vi "MapAction.vi"(2 "error in (no error)":errorcluster, 3 "Action":enum16{"Remove", "Mark", "Clear All"}(ring), 4 "Id":string, 5 "EpiWrapper in":refnum<class "EpiWrapper.lvclass">) -> (0 "error out":errorcluster, 1 "EpiWrapper out":refnum<class "EpiWrapper.lvclass">)   [LabVIEW 2012, in "EpiWrapper.lvclass"]
uses:
  EpiWrapper.lvclass
  EpiWrapper.lvclass/EpiWrapper.ctl
  Controls/CurrentPad.ctl
  Controls/PadArea.ctl
  Controls/Pad.ctl
  Controls/SelectedPads.ctl
  PadLookupVar.vi
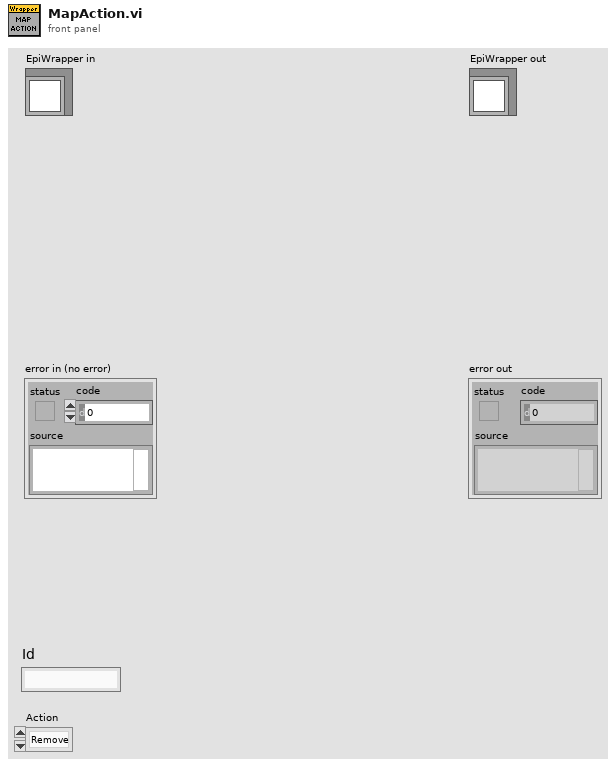
[diagram p1: front panel]
types:
  T1 = typedef "Pad.ctl" = cluster{"Coords":cluster{"Horizontal":sgl, "Vertical":sgl}, "radius":i32, "Tested":bool, "Selected":bool, "Id":string}
  T2 = typedef "MeasureControl.ctl" = cluster{"Graph":cluster{"Y":dbl[], "Y":dbl[]}[], "Pass":bool, "Fail":bool, "Measure":bool, "Wafer Area":T3, "TestData":T4, "Pad":string}
  T3 = typedef "PadArea.ctl" = enum16{"CenterA", "CenterB", "CenterC", "CenterD", "L", "R", "T", "G"}
  T4 = typedef "TestData.ctl" = cluster{"20mA Data":T5, "50mA Data ":T5}
  T5 = typedef "Measurement.ctl" = cluster{"Area":string, "Pad":string, "Current,mA":dbl, "Power":dbl, "WL":dbl, "Voltage":dbl, "Knee Current":dbl, "Reverse":dbl}
  T6 = typedef "SelectedPads.ctl" = T1[]
  T7 = typedef "CurrentPad.ctl" = cluster{"Coords":cluster{"Horizontal":sgl, "Vertical":sgl}, "radius":i32, "Tested":bool, "Selected":bool, "Pad":string, "PadArea":T8}
  T8 = typedef "PadArea.ctl" = enum16{"A", "B", "C", "D", "L", "R", "T", "G"}
  T9 = typedef "MapPOS.ctl" = cluster{"Coords":cluster{"Horizontal":sgl, "Vertical":sgl}, "radius":i32, "state":bool, "Id":string}[]
  T10 = typedef "PadLookup.ctl" = cluster{"A":T11, "B":T11, "C":T11, "D":T11, "L":T11, "R":T11, "T":T11, "G":T11}
  T11 = typedef "PadLookupItem.ctl" = cluster{"PadArea":T8, string[]}
  T12 = typedef "MeasureControl.ctl" = cluster{"Graph":cluster{"Y":dbl[], "Y":dbl[]}[], "Pass":bool, "Fail":bool, "Measure":bool, "Wafer Area":T8, "TestData":T4, "Pad":string}
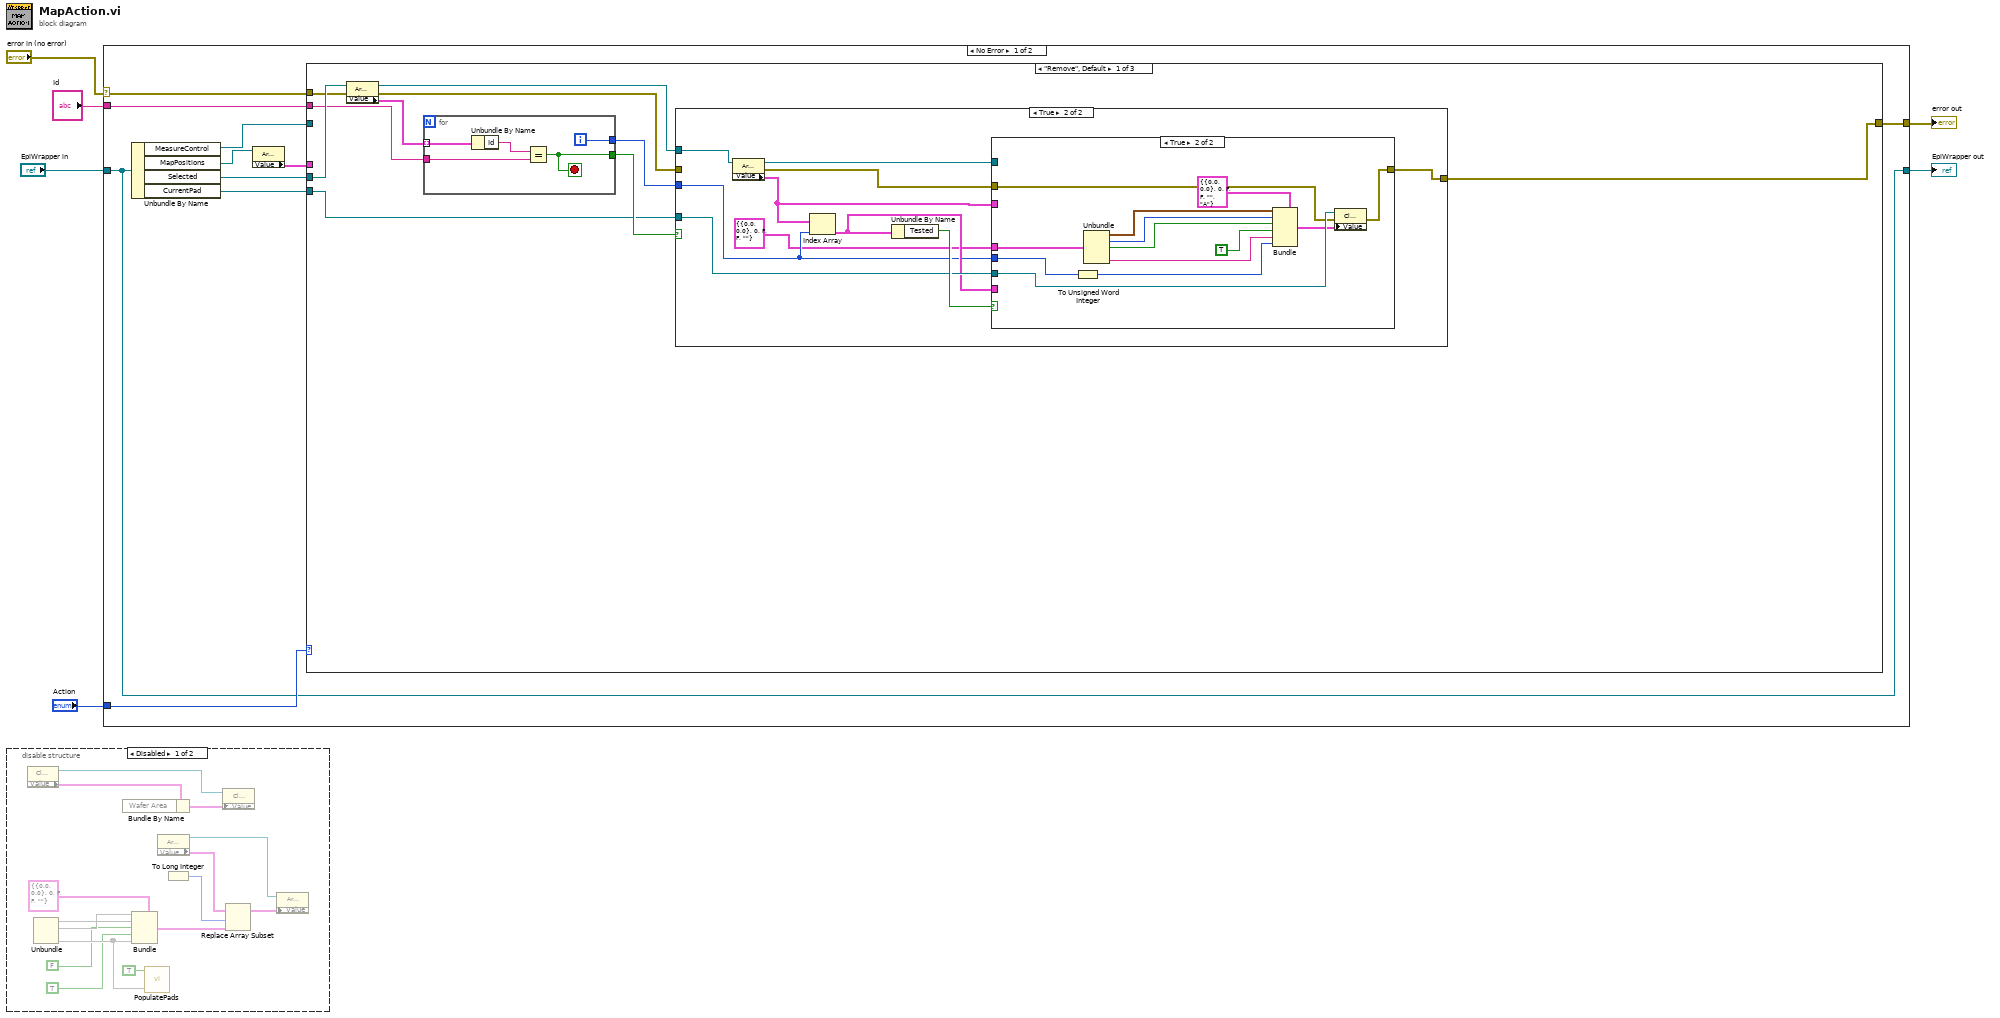
[diagram p0: block diagram]
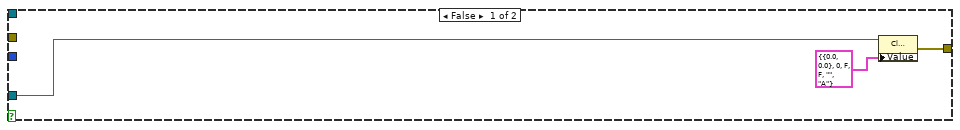
[diagram p3: hidden frame]
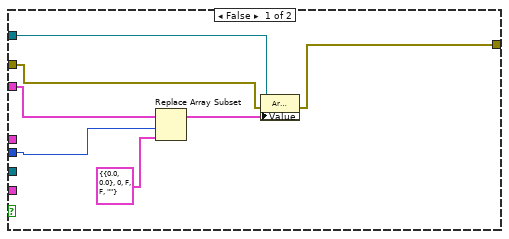
[diagram p4: hidden frame]
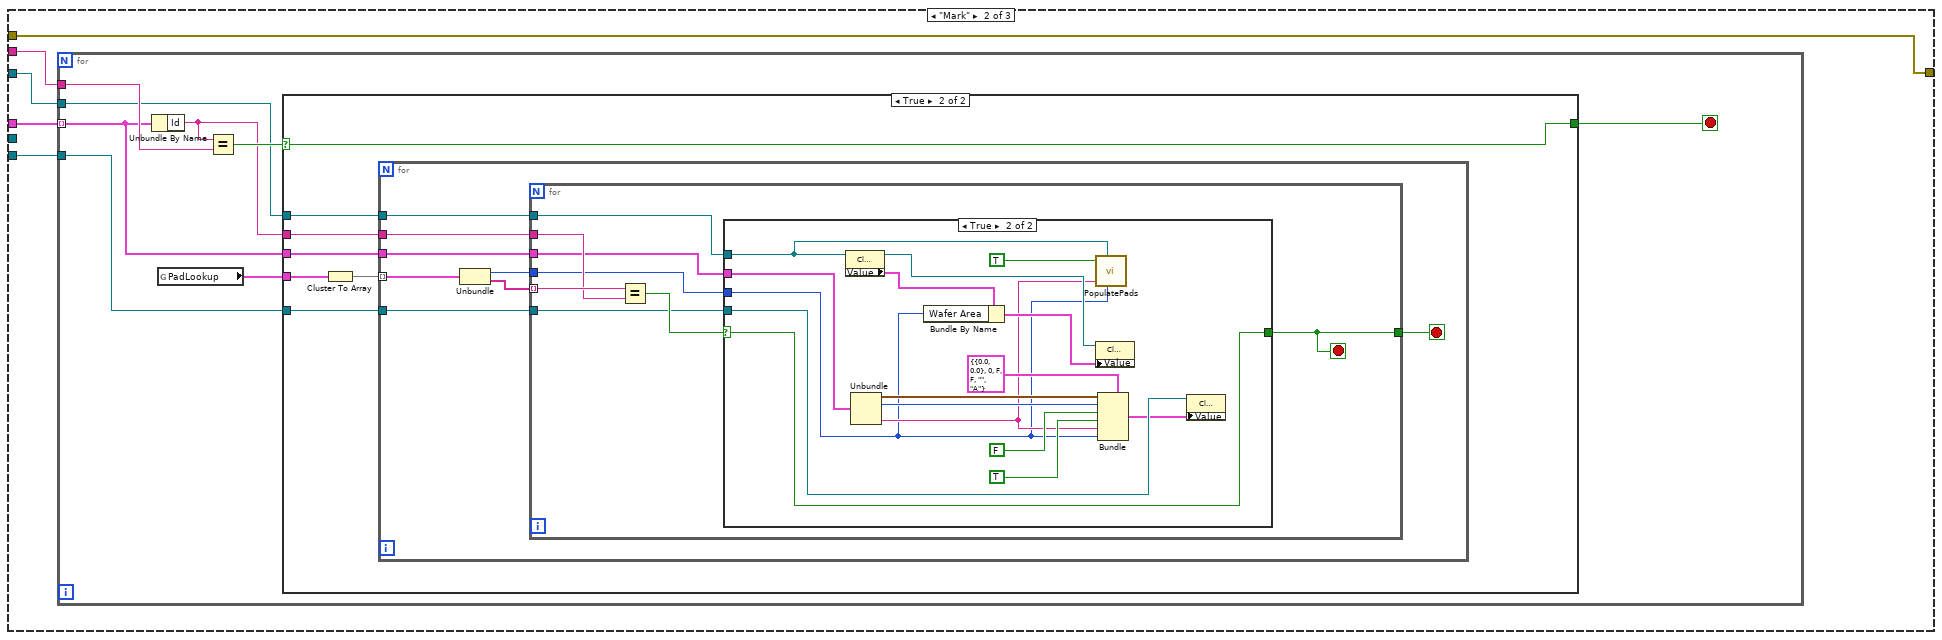
[diagram p5: hidden frame]
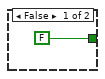
[diagram p6: hidden frame]
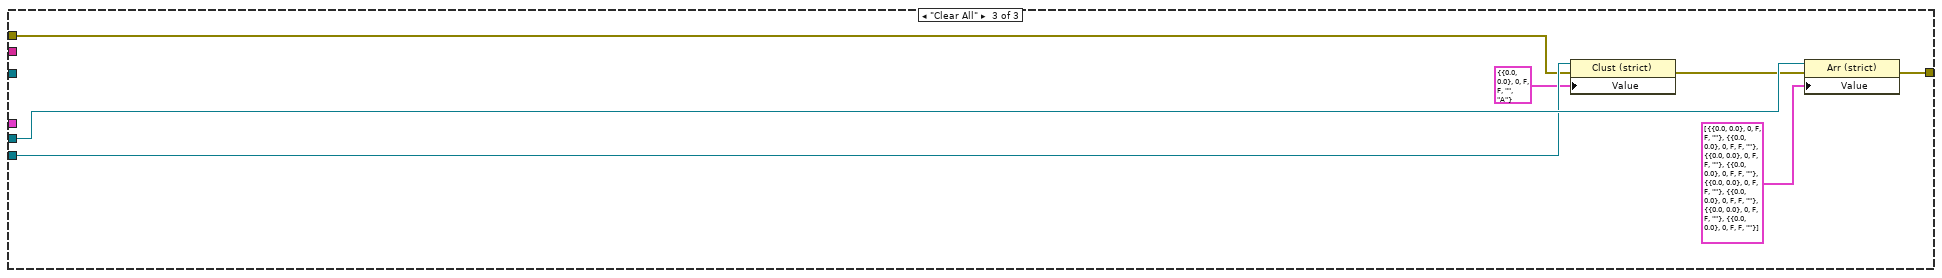
[diagram p8: hidden frame]
diagram:
  n1 = disable-structure shown="Disabled" {
    frame Disabled {
      n2 = property class="Clust (strict)"() -> (reference out=w18:refnum<vi>, "Value"=w17:T2)  [unwired: 2 in, 1 out]
      n3 = Unbundle() -> ("Coords"=w11, "radius"=w13, "Id"=w20)  [unwired: 1 in, 1 out]
      n4 = Bundle By Name(cluster=w17) -> (w19:T2)  [unwired: 1 in]
      n5 = Bundle(cluster=T1 {"Coords"={"Horizontal"=0.0, "Vertical"=0.0}, "radius"=0, "Tested"=FALSE, "Selected"=FALSE, "Id"=""} ("new element/subarray"), "Coords"=w11, "radius"=w13, "Tested"=FALSE, "Selected"=TRUE, "Id"=w20) -> (w14:T1)
      n6 = call "PopulatePads.vi"("Set Pad?"=TRUE, "Pad"=w20) -> ()  [unwired: 4 in]
      n7 = property class="Arr (strict)"() -> (reference out=w7:refnum<vi>, "Value"=w8:T6)  [unwired: 2 in, 1 out]
      n8 = To Long Integer() -> (32bit integer=w16:i32)  [unwired: 1 in]
      n9 = property class="Clust (strict)"(reference=w18, "Value"=w19) -> ()  [unwired: 1 in, 2 out]
      n10 = Replace Array Subset(array=w8, new element=w14, index=w16) -> (w15:T6)
      n11 = property class="Arr (strict)"(reference=w7, "Value"=w15) -> ()  [unwired: 1 in, 2 out]
    }
    frame Enabled {
    }
  }
  n12 = case shown="No Error" "error in (no error)" {
    selector: "error in (no error)" -> [w24 w142]
    tunnel: [w23 w142] -> w5
    tunnel: [w25 w141] -> w3
    tunnel: "EpiWrapper in" -> [w25 w141]
    tunnel: "Id" -> [w27 _]
    tunnel: "Action" -> [w26 _]
    frame No Error {
      n13 = Unbundle By Name(w25) -> ("MeasureControl"=w28:refnum<vi>, "MapPositions"=w29:refnum<vi>, "Selected"=w30:refnum<vi>, "CurrentPad"=w22:refnum<vi>)
      n14 = property class="Arr (strict)"(reference=w29) -> ("Value"=w31:T9)  [unwired: 1 in, 2 out]
      n15 = case shown="\"Remove\", Default" w26 {
        tunnel: w31 -> [_ w84 _]
        tunnel: w27 -> [w39 w83 _]
        tunnel: w30 -> [w41 _ w140]
        tunnel: w28 -> [_ w82 _]
        tunnel: w24 -> [w34 w81 w134]
        tunnel: [w32 w81 w138] -> w23
        tunnel: w22 -> [w35 w80 w137]
        frame "Remove", Default {
          n16 = property class="Arr (strict)"(reference=w41, error in=w34) -> (reference out=w36:refnum<vi>, error out=w33:errorcluster, "Value"=w40:T6)
          n17 = for {
            tunnel: w40 -> [w78] mode=indexing
            tunnel: w39 -> [w79]
            tunnel: [w75] -> w37
            tunnel: [w76] -> w38
            i -> [w75]
            stop <- w76 stop-if-true
            n18 = Unbundle By Name(w78) -> ("Id"=w77:string)
            n19 = Equal?(x=w77, y=w79) -> (x = y?=w76:bool)
          }
          n20 = case shown="True" w38 {
            tunnel: w37 -> [_ w51]
            tunnel: w36 -> [_ w48]
            tunnel: w35 -> [w44 w53]
            tunnel: [w42 w50] -> w32
            tunnel: w33 -> [_ _]
            frame False {
              n21 = property class="Clust (strict)"(reference=w44, "Value"=T7 {"Coords"={"Horizontal"=0.0, "Vertical"=0.0}, "radius"=0, "Tested"=FALSE, "Selected"=FALSE, "Pad"="", "PadArea"=enum."A"}) -> (error out=w42:errorcluster)  [unwired: 1 in, 1 out]
            }
            frame True {
              n22 = property class="Arr (strict)"(reference=w48) -> (reference out=w46:refnum<vi>, error out=w47:errorcluster, "Value"=w45:T6)  [unwired: 1 in]
              n23 = Index Array(array=w45, index=w51) -> (element=w52:T1)
              n24 = Unbundle By Name(w52) -> ("Tested"=w54:bool)
              n25 = case shown="True" w54 {
                tunnel: w53 -> [_ w74]
                tunnel: w52 -> [_ _]
                tunnel: T1 {"Coords"={"Horizontal"=0.0, "Vertical"=0.0}, "radius"=0, "Tested"=FALSE, "Selected"=FALSE, "Id"=""} ("new element/subarray") -> [_ w68]
                tunnel: w51 -> [w56 w65]
                tunnel: [w60 w63] -> w50
                tunnel: w47 -> [w59 w62]
                tunnel: w46 -> [w58 _]
                tunnel: w45 -> [w57 _]
                frame False {
                  n26 = Replace Array Subset(array=w57, new element=T1 {"Coords"={"Horizontal"=0.0, "Vertical"=0.0}, "radius"=0, "Tested"=FALSE, "Selected"=FALSE, "Id"=""} ("new element/subarray"), index=w56) -> (w61:T6)
                  n27 = property class="Arr (strict)"(reference=w58, error in=w59, "Value"=w61) -> (error out=w60:errorcluster)  [unwired: 1 out]
                }
                frame True {
                  n28 = To Unsigned Word Integer(number=w65) -> (unsigned 16bit integer=w64:u16)
                  n29 = Unbundle(w68) -> ("Coords"=w73:cluster{"Horizontal":sgl, "Vertical":sgl}, "radius"=w72:i32, "Tested"=w71:bool, "Id"=w69:string)  [unwired: 1 out]
                  n30 = Bundle(cluster=T7 {"Coords"={"Horizontal"=0.0, "Vertical"=0.0}, "radius"=0, "Tested"=FALSE, "Selected"=FALSE, "Pad"="", "PadArea"=enum."A"} ("Value"), "Coords"=w73, "radius"=w72, "Tested"=w71, "Selected"=TRUE, "Pad"=w69, "PadArea"=w64) -> (w66:T7)
                  n31 = property class="Clust (strict)"(reference=w74, error in=w62, "Value"=w66) -> (error out=w63:errorcluster)  [unwired: 1 out]
                }
              }
            }
          }
        }
        frame "Mark" {
          n32 = for {
            tunnel: w84 -> [w88] mode=indexing
            tunnel: w83 -> [w92]
            tunnel: w82 -> [w87]
            tunnel: w80 -> [w85]
            stop <- w90 stop-if-true
            n33 = Unbundle By Name(w88) -> ("Id"=w89:string)
            n34 = global read "PadLookupVar.vi" "PadLookup"() -> (w86:T10)
            n35 = Equal?(x=w89, y=w92) -> (x = y?=w91:bool)
            n36 = case shown="True" w91 {
              selector: w91 -> [_ w100]
              tunnel: [FALSE w100] -> w90
              tunnel: w89 -> [_ w98]
              tunnel: w88 -> [_ w97]
              tunnel: w87 -> [_ w96]
              tunnel: w86 -> [_ w95]
              tunnel: w85 -> [_ w94]
              frame False {
              }
              frame True {
                n37 = Cluster To Array(cluster=w95) -> (array=w99:T11[])
                n38 = for {
                  tunnel: w99 -> [w105] mode=indexing
                  tunnel: w98 -> [w107]
                  tunnel: w97 -> [w104]
                  tunnel: w96 -> [w102]
                  tunnel: w94 -> [w101]
                  stop <- w103 stop-if-true
                  n39 = Unbundle(w105) -> ("PadArea"=w106:T8, w108:string[])
                  n40 = for {
                    tunnel: w108 -> [w116] mode=indexing
                    tunnel: w107 -> [w115]
                    tunnel: w106 -> [w113]
                    tunnel: w104 -> [w112]
                    tunnel: [w111] -> w103
                    tunnel: w102 -> [w110]
                    tunnel: w101 -> [w109]
                    stop <- w111 stop-if-true
                    n41 = Equal?(x=w116, y=w115) -> (x = y?=w114:bool)
                    n42 = case shown="True" w114 {
                      selector: w114 -> [w117 w132]
                      tunnel: w113 -> [_ w118]
                      tunnel: w112 -> [_ w133]
                      tunnel: [w117 w132] -> w111
                      tunnel: w110 -> [_ w128]
                      tunnel: w109 -> [_ w122]
                      frame False {
                      }
                      frame True {
                        n43 = property class="Clust (strict)"(reference=w128) -> (reference out=w130:refnum<vi>, "Value"=w131:T12)  [unwired: 1 in, 1 out]
                        n44 = Unbundle(w133) -> ("Coords"=w125:cluster{"Horizontal":sgl, "Vertical":sgl}, "radius"=w124:i32, "Id"=w119:string)  [unwired: 1 out]
                        n45 = Bundle By Name(cluster=w131, "Wafer Area"=w118) -> (w129:T12)
                        n46 = call "PopulatePads.vi"("Set Pad?"=TRUE, "MeasureControl"=w128, "Pad"=w119, "PadArea"=w118) -> ()  [unwired: 2 in]
                        n47 = property class="Clust (strict)"(reference=w130, "Value"=w129) -> ()  [unwired: 1 in, 2 out]
                        n48 = Bundle(cluster=T7 {"Coords"={"Horizontal"=0.0, "Vertical"=0.0}, "radius"=0, "Tested"=FALSE, "Selected"=FALSE, "Pad"="", "PadArea"=enum."A"} ("Value"), "Coords"=w125, "radius"=w124, "Tested"=FALSE, "Selected"=TRUE, "Pad"=w119, "PadArea"=w118) -> (w121:T7)
                        n49 = property class="Clust (strict)"(reference=w122, "Value"=w121) -> ()  [unwired: 1 in, 2 out]
                      }
                    }
                  }
                }
              }
            }
          }
        }
        frame "Clear All" {
          n50 = property class="Clust (strict)"(reference=w137, error in=w134, "Value"=T7 {"Coords"={"Horizontal"=0.0, "Vertical"=0.0}, "radius"=0, "Tested"=FALSE, "Selected"=FALSE, "Pad"="", "PadArea"=enum."A"}) -> (error out=w135:errorcluster)  [unwired: 1 out]
          n51 = property class="Arr (strict)"(reference=w140, error in=w135, "Value"=T6 [{"Coords"={"Horizontal"=0.0, "Vertical"=0.0}, "radius"=0, "Tested"=FALSE, "Selected"=FALSE, "Id"=""}, {"Coords"={"Horizontal"=0.0, "Vertical"=0.0}, "radius"=0, "Tested"=FALSE, "Selected"=FALSE, "Id"=""}, {"Coords"={"Horizontal"=0.0, "Vertical"=0.0}, "radius"=0, "Tested"=FALSE, "Selected"=FALSE, "Id"=""}, {"Coords"={"Horizontal"=0.0, "Vertical"=0.0}, "radius"=0, "Tested"=FALSE, "Selected"=FALSE, "Id"=""}, {"Coords"={"Horizontal"=0.0, "Vertical"=0.0}, "radius"=0, "Tested"=FALSE, "Selected"=FALSE, "Id"=""}, {"Coords"={"Horizontal"=0.0, "Vertical"=0.0}, "radius"=0, "Tested"=FALSE, "Selected"=FALSE, "Id"=""}, {"Coords"={"Horizontal"=0.0, "Vertical"=0.0}, "radius"=0, "Tested"=FALSE, "Selected"=FALSE, "Id"=""}, {"Coords"={"Horizontal"=0.0, "Vertical"=0.0}, "radius"=0, "Tested"=FALSE, "Selected"=FALSE, "Id"=""}] ("WaferPads 2")) -> (error out=w138:errorcluster)  [unwired: 1 out]
        }
      }
    }
    frame Error {
    }
  }
  "error out" <- w5
  "EpiWrapper out" <- w3
